vi "Logger Stopped.vi"(8 "error in (no error)":errorcluster, 10 "Logger Stopped":T1, 11 "Historian Logger in":refnum<class "Historian Logger.lvclass">) -> (0 "error out":errorcluster, 3 "Historian Logger out":refnum<class "Historian Logger.lvclass">)   [LabVIEW 2020, in "VolatusHistorian.lvlib" / "Historian Logger.lvclass"]
uses:
  Historian Logger.lvclass
  C:/dev/lv20CE/relink/lv-volatus/Volatus/Module/Module.lvclass
  VolatusData/Logger Stopped.ctl
  Volatus/Module/Module.lvclass/Module.ctl
  Historian Logger.lvclass/Historian Logger.ctl
  VolatusData/Logger State.ctl
  VolatusData/VolatusData.lvlib
  Volatus/Module/Module.lvclass
  lv-cdm/CDM-Config/CDM-Config.lvlib
  lv-cdm/CDM-Config/Format.ctl
  lv-cdm/CDM-Config/Precision.ctl
  lv-cdm/CDM-Config/Timezone.ctl
  lv-cdm/CDM-Config/ISO8601 Config.ctl
  C:/dev/lv20CE/relink/lv-volatus/VolatusHistorian/Historian Logger/Historian Logger.lvclass
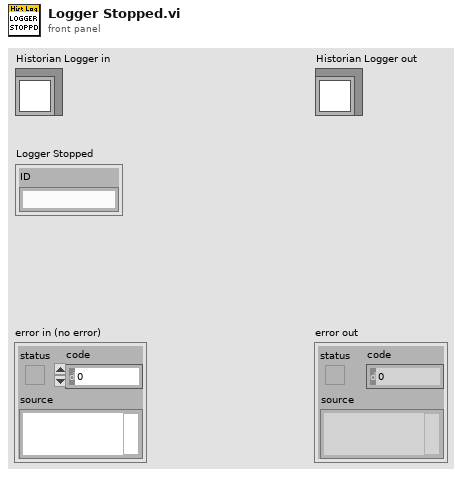
[diagram p1: front panel]
types:
  T1 = typedef "VolatusData.lvlib/Logger Stopped.ctl" = cluster{"ID":string}
  T2 = typedef "CDM-Config.lvlib/ISO8601 Config.ctl" = cluster{"Format":T3, "Precision":T4, "Timezone":T5}
  T3 = typedef "CDM-Config.lvlib/Format.ctl" = enum16{"Extended", "Basic"}
  T4 = typedef "CDM-Config.lvlib/Precision.ctl" = enum16{"Millisecond", "Second", "Minute", "Hour", "Day"}
  T5 = typedef "CDM-Config.lvlib/Timezone.ctl" = enum16{"UTC", "Local"}
  T6 = typedef "VolatusData.lvlib/Logger State.ctl" = enum16{"Unknown", "Idle", "Preparing", "Ready", "Logging", "Stopping"}
  T7 = typedef "VolatusHistorian.lvlib/Historian Logger.lvclass/Group Info.ctl" = cluster{"Buffer":refnum<class "Group Buffer DBL.lvclass">, "Logger":refnum<class "MessageQ.lvclass">, "Group":refnum<class "Group.lvclass">, "Last Timestamp":dbl, "State":T6}
  T8 = typedef "VolatusData.lvlib/Prepare Log.ctl" = cluster{"Folder":path, "Series":string}
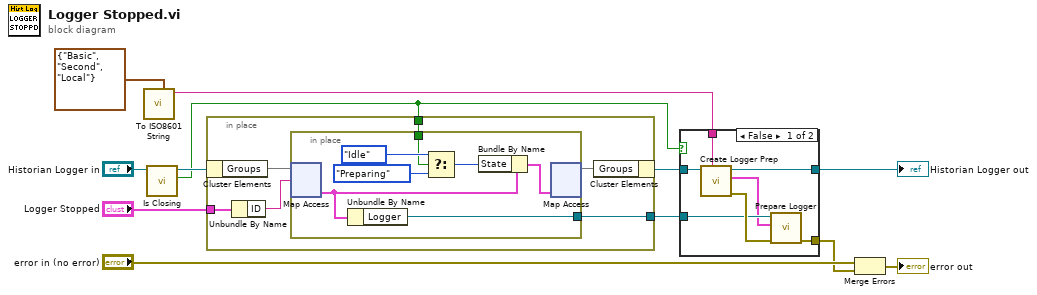
[diagram p0: block diagram]
diagram:
  n1 = call "To ISO8601 String.vi"("Format Config"=T2 {"Format"=enum."Basic", "Precision"=enum."Second", "Timezone"=enum."Local"}) -> ("ISO 8601"=w1:string)  [unwired: 10 in]
  n2 = call "Is Closing.vi"("Module in"="Historian Logger in") -> ("Is Closing"=w3:bool, "Module out"=w4:refnum<class "Historian Logger.lvclass">)  [unwired: 9 in]
  n3 = in-place {
    in-place-border: "Logger Stopped" -> [w18]
    in-place-border: [w14] -> w8
    in-place-border: w3 -> [w13]
    n4 = in-place-cluster #1(w4) -> ("Groups"=w17:map{string, T7})
    n5 = Unbundle By Name(w18) -> ("ID"=w16:string)
    n6 = in-place {
      in-place-border: [w23] -> w14
      in-place-border: w13 -> [w19]
      n7 = in-place-map #2(w17, w16) -> (w24:T7)  [unwired: 1 in, 1 out]
      n8 = Unbundle By Name(w24) -> ("Logger"=w23:refnum<class "MessageQ.lvclass">)
      n9 = Select(t=Logger_State."Idle" ("State"), s=w19, f=Logger_State."Preparing") -> (s? t:f=w20:T6)
      n10 = Bundle By Name(cluster=w24, "State"=w20) -> (w25:T7)
      n11 = in-place-map #2(w25) -> (w15:map{string, T7})  [unwired: 1 in, 2 out]
    }
    n12 = in-place-cluster #1("Groups"=w15) -> (w10:refnum<class "Historian Logger.lvclass">)
  }
  n13 = case shown="False" w3 {
    tunnel: w10 -> [w31 w33]
    tunnel: w8 -> [w30 _]
    tunnel: [w29 w33] -> w7
    tunnel: [w27 _] -> w6
    tunnel: w1 -> [w26 _]
    frame False {
      n14 = call "Create Logger Prep.vi"("Timestamp"=w26, "Historian Logger in"=w31) -> ("error out"=w32:errorcluster, "Logger Info"=w28:T8, "Historian Logger out"=w29:refnum<class "Historian Logger.lvclass">)  [unwired: 7 in]
      n15 = call "Prepare Logger.vi"("error in (no error)"=w32, "Prepare Log"=w28, "MsgQ in"=w30) -> ("error out"=w27:errorcluster)  [unwired: 7 in, 1 out]
    }
    frame True {
    }
  }
  "Historian Logger out" <- w7
  n16 = Merge Errors("error in (no error)", w6) -> (→"error out":errorcluster)
